vi "Is Path to Actor.vi"(8 "error in (no error)":errorcluster, 10 "Target":refnum<vi>, 11 "Path":path) -> (0 "error out":errorcluster, 1 "Default Actor Path":path, 2 "Is Path to Actor?":bool)   [LabVIEW 2020, in "Message Maker.lvlib"]
uses:
  Message Maker.lvlib
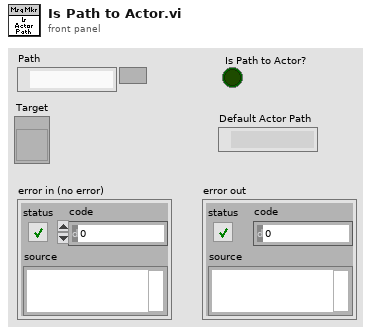
[diagram p1: front panel]
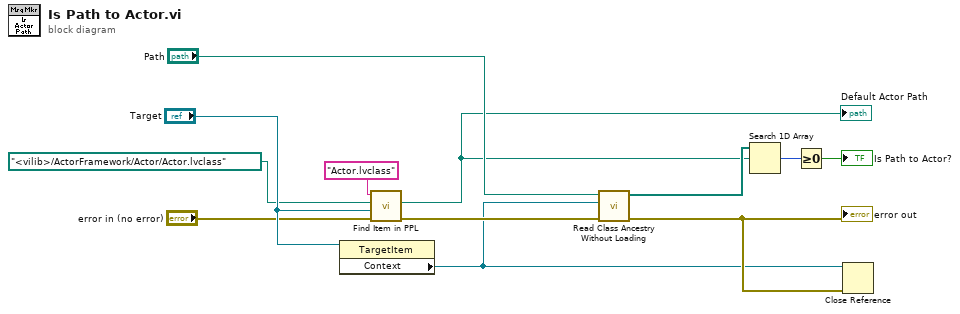
[diagram p0: block diagram]
diagram:
  n1 = property class="TargetItem"(reference="Target") -> ("Context"=w3:refnum<vi>)  [unwired: 1 in, 2 out]
  n2 = call "Find Item in PPL.vi"("error in (no error)"="error in (no error)", "Target"="Target", "default path"=path "<vilib>/ActorFramework/Actor/Actor.lvclass", "qualified name"="Actor.lvclass") -> ("error out"=w8:errorcluster, "item path out"=w7:path)  [unwired: 5 in, 1 out]
  "Default Actor Path" <- w7
  n3 = call <vilib>:"Read Class Ancestry Without Loading.vi"("error in (no error)"=w8, "App Reference (this app)"=w3, "LabVIEW Class Path"="Path") -> ("error out"=w4:errorcluster, "Class Ancestry"=w10:path[])  [unwired: 7 in]
  "error out" <- w4
  n4 = Search 1D Array(1D array=w10, element=w7) -> (index of element=w12:i32)  [unwired: 1 in]
  n5 = Greater Or Equal To 0?(x=w12) -> (x >= 0?=→"Is Path to Actor?":bool)
  n6 = Close Reference(reference=w3, error in (no error)=w4) -> ()  [unwired: 1 out]
